vi "Autonomous Independent (Spencer Scott's conflicted copy 2017-03-24).vi"() -> ()   [LabVIEW 2016]
doc: "This VI is called when autonomous begins, and will automatically be terminated when autonomous ends. You can carry out timed or sensor driven robot movement independently without needing to return to the caller."
uses:
  Control 1.ctl
  <vilib>/Rock Robotics/Network Tables/NT Read String.vi
  <vilib>/Rock Robotics/Network Tables/NT Write String.vi
  Robot Global Data.vi
panel:
  in  "Drive PID":T1={"proportional gain (Kc)"=0.08, "integral time (Ti, min)"=0.0, "derivative time (Td, min)"=0.0} {"derivative time (Td, min)" format="%.3f"; "integral time (Ti, min)" format="%.3f"; "proportional gain (Kc)" format="%.3f"}
  # "Be sure to right-click and choose Data Operations>>Make Current Value default if you want to save the array values with the VI"
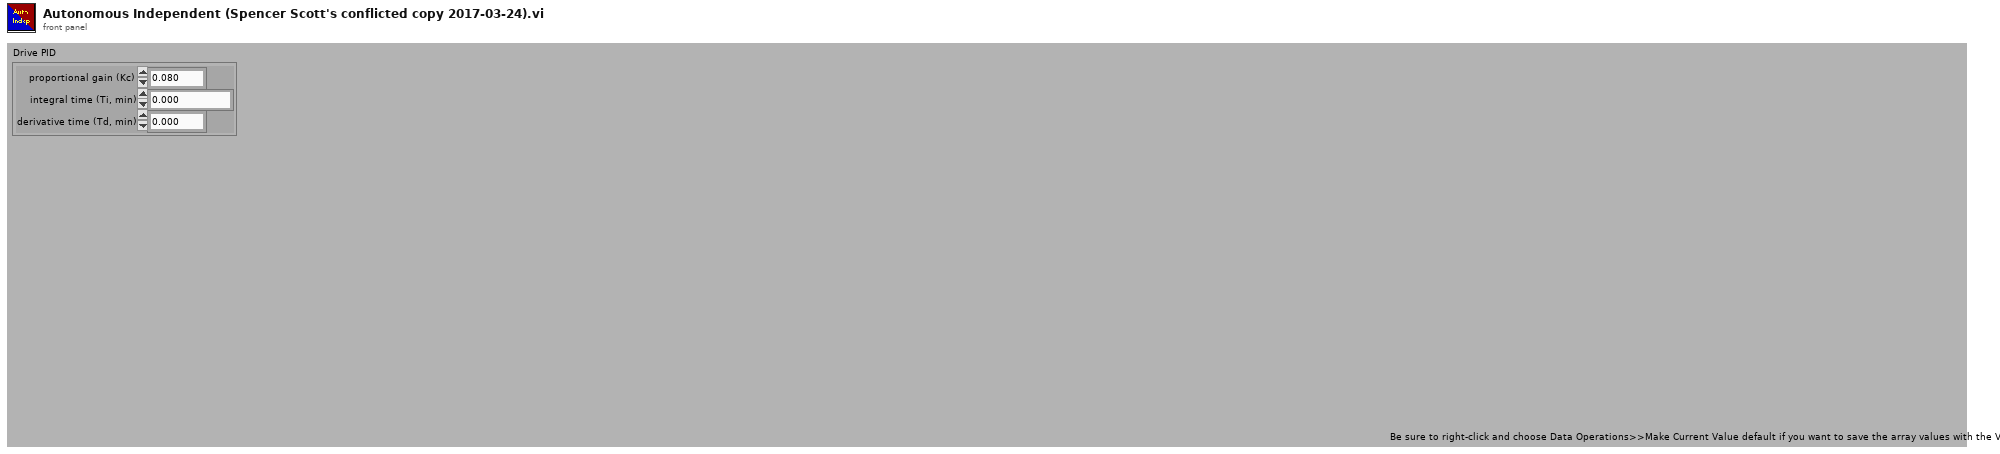
[diagram p1: front panel]
types:
  T1 = cluster{"proportional gain (Kc)":dbl, "integral time (Ti, min)":dbl, "derivative time (Td, min)":dbl}
  T2 = typedef "WPI_GyroDevRef.ctl" = cluster{"DevStatus":errorcluster, "Analog Channel":T3, "Offset":dbl, "Gain (VoltsPerDegree/Second)":dbl, "Gyro Type":enum16{"Analog", "XRS450"}, "Handle":i32, "SPI Bus":T4, "Device Found":bool, "Sample Rate":dbl, "Calibrate On Open":bool}
  T3 = typedef "FPGA_AIChannel.ctl" = enum8{"AI 0", "AI 1", "AI 2", "AI 3", "AI MXP 0", "AI MXP 1", "AI MXP 2", "AI MXP 3", "Invalid"}
  T4 = typedef "spi_bus.ctl" = enum16{"SPI On-Board, CS0", "SPI On-Board, CS1", "SPI On-Board, CS2", "SPI On-Board, CS3", "SPI MXP", "Invalid"}
  T5 = typedef "WPI_DriverStationAllianceInfo.ctl" = enum16{"Red", "Blue", "Invalid"}
  T6 = typedef "Control 1.ctl" = u32
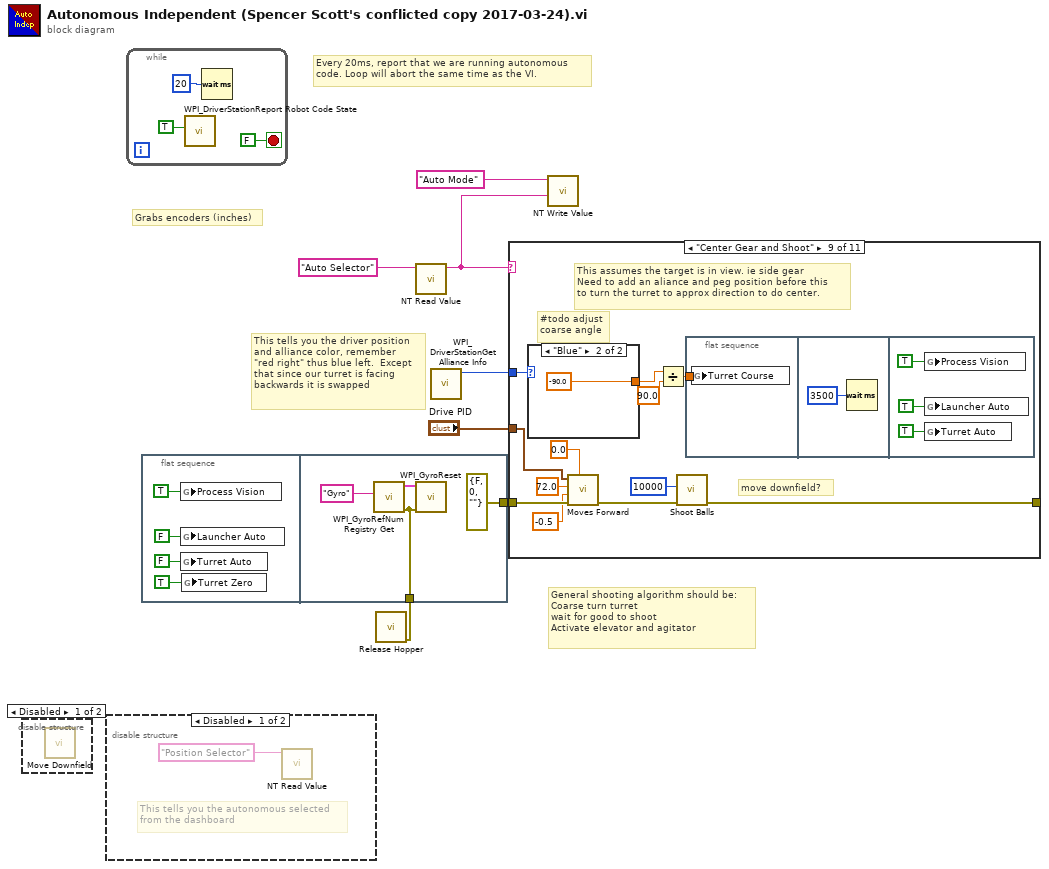
[diagram p0: block diagram]
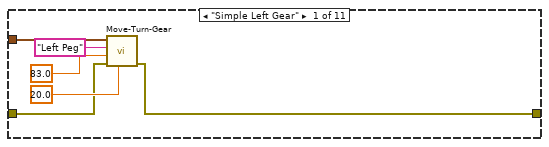
[diagram p4: hidden frame]
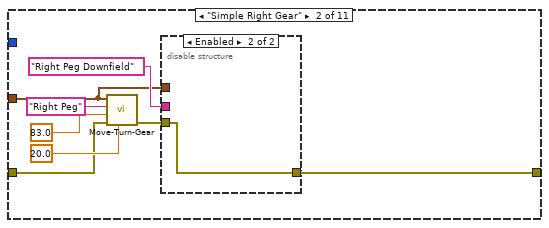
[diagram p5: hidden frame]
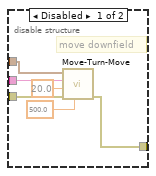
[diagram p6: hidden frame]
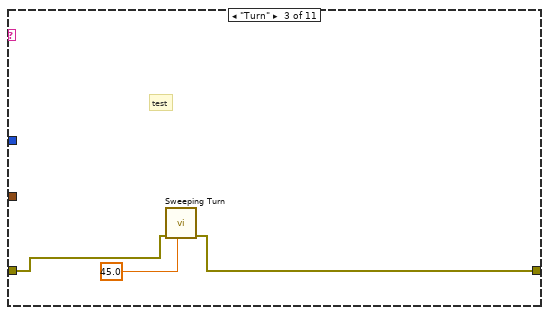
[diagram p7: hidden frame]
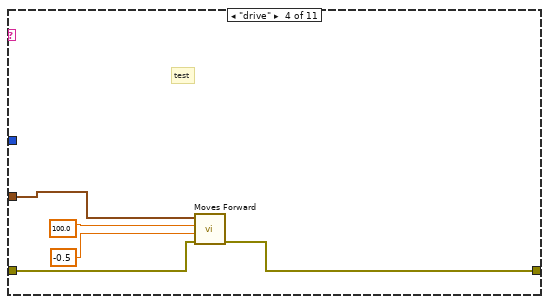
[diagram p8: hidden frame]
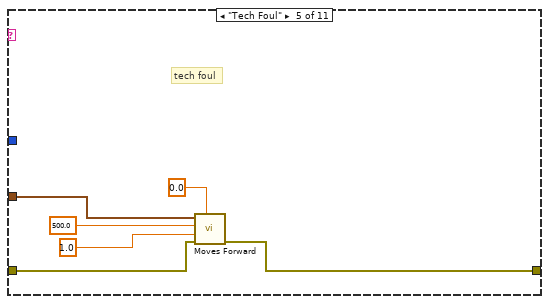
[diagram p9: hidden frame]
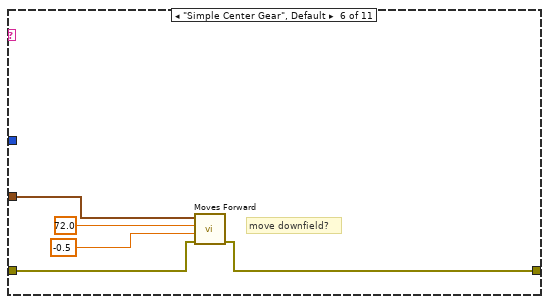
[diagram p10: hidden frame]
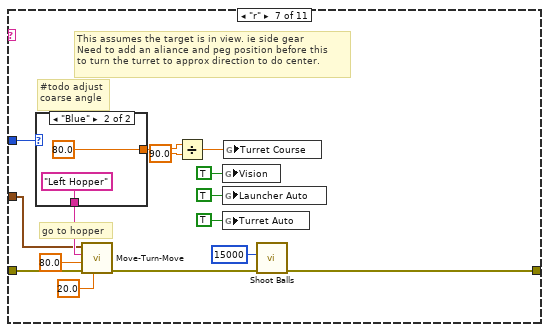
[diagram p11: hidden frame]
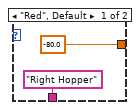
[diagram p12: hidden frame]
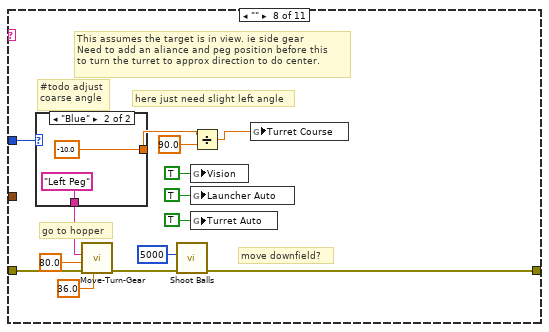
[diagram p13: hidden frame]
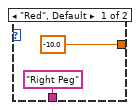
[diagram p14: hidden frame]
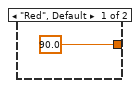
[diagram p15: hidden frame]
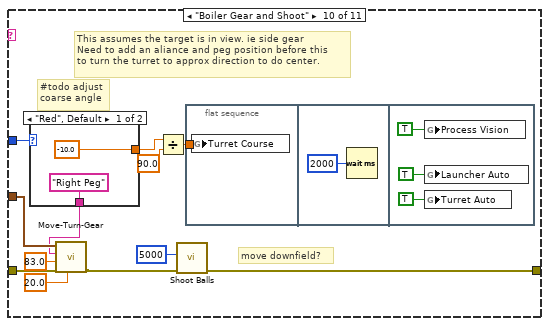
[diagram p16: hidden frame]
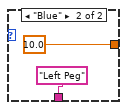
[diagram p17: hidden frame]
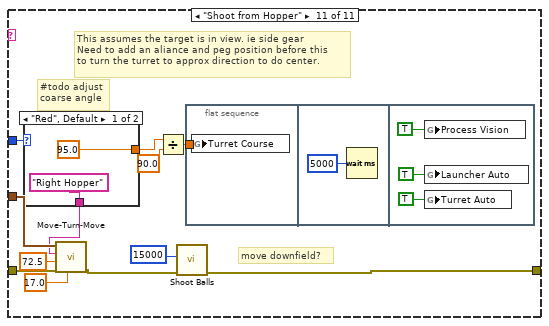
[diagram p18: hidden frame]
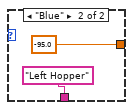
[diagram p19: hidden frame]
diagram:
  # "General shooting algorithm should be:\nCoarse turn turret\nwait for good to shoot\nActivate elevator and agitator"
  # "Every 20ms, report that we are running autonomous\ncode. Loop will abort the same time as the VI."
  # "This tells you the driver position\nand alliance color, remember\n\"red right\" thus blue left.  Except\nthat since our turret is facing\nbackwards it is swapped"
  # "Grabs encoders (inches)"
  n1 = disable-structure shown="Disabled" {
    frame Disabled {
      n2 = call "Move Downfield.vi"() -> ()  [unwired: 11 in, 1 out]
    }
    frame Enabled {
    }
  }
  n3 = disable-structure shown="Disabled" {
    frame Disabled {
      # "This tells you the autonomous selected\nfrom the dashboard"
      n4 = call-poly <vilib>:"NT Read Value.vi"("Name"="Position Selector") -> ()  [unwired: 9 in, 2 out]
    }
    frame Enabled {
    }
  }
  n5 = while {
    stop <- FALSE stop-if-true
    n6 = call <vilib>:"WPI_DriverStationReport Robot Code State.vi"("Autonomous"=TRUE) -> ()  [unwired: 10 in, 1 out]
    n7 = Wait (ms)(milliseconds to wait=u32 20) -> ()  [unwired: 1 out]
  }
  n8 = flat-sequence {
    tunnel: [w17] -> w3
    tunnel: [errorcluster {"status"=FALSE, "code"=0, "source"=""} ("error out")] -> w1
    frame #0 {
      n9 = global write "Robot Global Data.vi" "Process Vision"(TRUE ("Launcher Auto")) -> ()
      n10 = global write "Robot Global Data.vi" "Launcher Auto"(FALSE ("Launcher Auto")) -> ()
      n11 = global write "Robot Global Data.vi" "Turret Auto"(FALSE ("Launcher Auto")) -> ()
      n12 = global write "Robot Global Data.vi" "Turret Zero"(TRUE ("Launcher Auto")) -> ()
    }
    frame #1 {
      n13 = call <vilib>:"WPI_GyroRefNum Registry Get.vi"("refnum name"="Gyro") -> ("error out"=w17:errorcluster, "GyroDevRef"=w19:T2)  [unwired: 9 in]
      n14 = call <vilib>:"WPI_GyroReset.vi"("error in"=w17, "GyroDevRef"=w19) -> ()  [unwired: 8 in, 2 out]
    }
  }
  n15 = call "Release Hopper.vi"("error in (no error)"=w3) -> ()  [unwired: 10 in, 1 out]
  n16 = call-poly <vilib>:"NT Read Value.vi"("Name"="Auto Selector") -> ("String"=w4:string)  [unwired: 9 in, 1 out]
  n17 = call <vilib>:"WPI_DriverStationGet Alliance Info.vi"() -> ("Alliance"=w2:T5)  [unwired: 11 out]
  n18 = case shown="\"Center Gear and Shoot\"" w4 {
    tunnel: "Drive PID" -> [w21 w27 _ w47 w53 w58 w60 _ w100 w117 w138]
    tunnel: w1 -> [w23 w31 w41 w48 w54 w59 w74 w92 w105 w121 w142]
    tunnel: [w20 w26 w43 w44 w51 w55 w73 w91 w108 w127 w148] -> _
    tunnel: w2 -> [_ _ _ _ _ _ w66 w84 w107 w126 w147]
    frame "Simple Left Gear" {
      n19 = call "Move-Turn-Gear.vi"("toGear"=20.0, "error in (no error)"=w23, "gearDistance"=83.0, "Position"="Left Peg", "PID gains"=w21) -> ("error out"=w20:errorcluster)  [unwired: 6 in]
    }
    frame "Simple Right Gear" {
      n20 = call "Move-Turn-Gear.vi"("toGear"=20.0, "error in (no error)"=w31, "gearDistance"=83.0, "Position"="Right Peg", "PID gains"=w27) -> ("error out"=w29:errorcluster)  [unwired: 6 in]
      n21 = disable-structure shown="Enabled" {
        disable-tunnel: w29 -> [w39 w40]
        disable-tunnel: "Right Peg Downfield" ("Position") -> [w38 _]
        disable-tunnel: w27 -> [w37 _]
        disable-tunnel: [w36 w40] -> w26
        frame Disabled {
          # "move downfield"
          n22 = call "Move-Turn-Move.vi"("toGear"=500.0, "error in (no error)"=w39, "gearDistance"=20.0, "Position"=w38, "PID gains"=w37) -> ("error out"=w36:errorcluster)  [unwired: 6 in]
        }
        frame Enabled {
        }
      }
    }
    frame "Turn" {
      # "test"
      n23 = call "Sweeping Turn.vi"("upper angle limit"=45.0 ("upper limit"), "error in"=w41) -> ("error out"=w43:errorcluster)  [unwired: 9 in]
    }
    frame "drive" {
      # "test"
      n24 = call "Moves Forward.vi"("error in (no error)"=w48, "Speed"=-0.5, "forwardDistance"=100.0, "PID gains"=w47) -> ("error out"=w44:errorcluster)  [unwired: 5 in, 2 out]
    }
    frame "Tech Foul" {
      # "tech foul"
      n25 = call "Moves Forward.vi"("yaw setpoint"=0.0, "error in (no error)"=w54, "Speed"=1.0, "forwardDistance"=500.0, "PID gains"=w53) -> ("error out"=w51:errorcluster)  [unwired: 4 in, 2 out]
    }
    frame "Simple Center Gear", Default {
      # "move downfield?"
      n26 = call "Moves Forward.vi"("error in (no error)"=w59, "Speed"=-0.5, "forwardDistance"=72.0, "PID gains"=w58) -> ("error out"=w55:errorcluster)  [unwired: 5 in, 2 out]
    }
    frame "r" {
      # "#todo adjust\ncoarse angle"
      # "This assumes the target is in view. ie side gear\nNeed to add an aliance and peg position before this\nto turn the turret to approx direction to do center."
      # "go to hopper"
      n27 = case shown="\"Blue\"" w66 {
        tunnel: [-80.0 80.0] -> w65
        tunnel: ["Right Hopper" ("Name") "Left Hopper" ("Name")] -> w63
        frame "Red", Default {
        }
        frame "Blue" {
        }
      }
      n28 = call "Move-Turn-Move.vi"("toGear"=20.0, "error in (no error)"=w74, "gearDistance"=80.0, "Position"=w63, "PID gains"=w60) -> ("error out"=w72:errorcluster)  [unwired: 6 in]
      n29 = Divide(x=w65, y=90.0) -> (x/y=w62:dbl)
      n30 = global write "Robot Global Data.vi" "Vision"(TRUE ("Launcher Auto")) -> ()
      n31 = global write "Robot Global Data.vi" "Launcher Auto"(TRUE ("Launcher Auto")) -> ()
      n32 = global write "Robot Global Data.vi" "Turret Auto"(TRUE ("Launcher Auto")) -> ()
      n33 = global write "Robot Global Data.vi" "Turret Course"(w62) -> ()
      n34 = call "Shoot Balls.vi"("error in (no error)"=w72, "milliseconds to shoot"=u32 15000) -> ("error out"=w73:errorcluster)  [unwired: 9 in]
    }
    frame "" {
      # "move downfield?"
      # "here just need slight left angle"
      # "#todo adjust\ncoarse angle"
      # "This assumes the target is in view. ie side gear\nNeed to add an aliance and peg position before this\nto turn the turret to approx direction to do center."
      # "go to hopper"
      n35 = case shown="\"Blue\"" w84 {
        tunnel: [-10.0 -10.0] -> w81
        tunnel: ["Right Peg" ("Name") "Left Peg" ("Name")] -> w82
        frame "Red", Default {
        }
        frame "Blue" {
        }
      }
      n36 = call "Move-Turn-Gear.vi"("toGear"=36.0, "error in (no error)"=w92, "gearDistance"=80.0, "Position"=w82) -> ("error out"=w90:errorcluster)  [unwired: 7 in]
      n37 = call "Shoot Balls.vi"("error in (no error)"=w90, "milliseconds to shoot"=u32 5000) -> ("error out"=w91:errorcluster)  [unwired: 9 in]
      n38 = global write "Robot Global Data.vi" "Vision"(TRUE ("Launcher Auto")) -> ()
      n39 = global write "Robot Global Data.vi" "Launcher Auto"(TRUE ("Launcher Auto")) -> ()
      n40 = global write "Robot Global Data.vi" "Turret Auto"(TRUE ("Launcher Auto")) -> ()
      n41 = Divide(x=w81, y=90.0) -> (x/y=w80:dbl)
      n42 = global write "Robot Global Data.vi" "Turret Course"(w80) -> ()
    }
    frame "Center Gear and Shoot" {
      # "move downfield?"
      # "#todo adjust\ncoarse angle"
      # "This assumes the target is in view. ie side gear\nNeed to add an aliance and peg position before this\nto turn the turret to approx direction to do center."
      n43 = case shown="\"Blue\"" w107 {
        tunnel: [90.0 -90.0] -> w98
        frame "Red", Default {
        }
        frame "Blue" {
        }
      }
      n44 = call "Moves Forward.vi"("yaw setpoint"=0.0, "error in (no error)"=w105, "Speed"=-0.5, "forwardDistance"=72.0, "PID gains"=w100) -> ("error out"=w104:errorcluster)  [unwired: 4 in, 2 out]
      n45 = Divide(x=w98, y=90.0) -> (x/y=w99:dbl)
      n46 = call "Shoot Balls.vi"("error in (no error)"=w104, "milliseconds to shoot"=T6 10000) -> ("error out"=w108:errorcluster)  [unwired: 9 in]
      n47 = flat-sequence {
        tunnel: w99 -> [w109]
        frame #0 {
          n48 = global write "Robot Global Data.vi" "Turret Course"(w109) -> ()
        }
        frame #1 {
          n49 = Wait (ms)(milliseconds to wait=u32 3500) -> ()  [unwired: 1 out]
        }
        frame #2 {
          n50 = global write "Robot Global Data.vi" "Process Vision"(TRUE ("Launcher Auto")) -> ()
          n51 = global write "Robot Global Data.vi" "Launcher Auto"(TRUE ("Launcher Auto")) -> ()
          n52 = global write "Robot Global Data.vi" "Turret Auto"(TRUE ("Launcher Auto")) -> ()
        }
      }
    }
    frame "Boiler Gear and Shoot" {
      # "move downfield?"
      # "#todo adjust\ncoarse angle"
      # "This assumes the target is in view. ie side gear\nNeed to add an aliance and peg position before this\nto turn the turret to approx direction to do center."
      n53 = case shown="\"Red\", Default" w126 {
        tunnel: [-10.0 10.0] -> w123
        tunnel: ["Right Peg" ("refnum name") "Left Peg" ("refnum name")] -> w116
        frame "Red", Default {
        }
        frame "Blue" {
        }
      }
      n54 = call "Move-Turn-Gear.vi"("toGear"=20.0, "error in (no error)"=w121, "gearDistance"=83.0, "Position"=w116, "PID gains"=w117) -> ("error out"=w120:errorcluster)  [unwired: 6 in]
      n55 = Divide(x=w123, y=90.0) -> (x/y=w124:dbl)
      n56 = call "Shoot Balls.vi"("error in (no error)"=w120, "milliseconds to shoot"=u32 5000) -> ("error out"=w127:errorcluster)  [unwired: 9 in]
      n57 = flat-sequence {
        tunnel: w124 -> [w128]
        frame #0 {
          n58 = global write "Robot Global Data.vi" "Turret Course"(w128) -> ()
        }
        frame #1 {
          n59 = Wait (ms)(milliseconds to wait=u32 2000) -> ()  [unwired: 1 out]
        }
        frame #2 {
          n60 = global write "Robot Global Data.vi" "Process Vision"(TRUE ("Launcher Auto")) -> ()
          n61 = global write "Robot Global Data.vi" "Launcher Auto"(TRUE ("Launcher Auto")) -> ()
          n62 = global write "Robot Global Data.vi" "Turret Auto"(TRUE ("Launcher Auto")) -> ()
        }
      }
    }
    frame "Shoot from Hopper" {
      # "move downfield?"
      # "#todo adjust\ncoarse angle"
      # "This assumes the target is in view. ie side gear\nNeed to add an aliance and peg position before this\nto turn the turret to approx direction to do center."
      n63 = case shown="\"Red\", Default" w147 {
        tunnel: [95.0 -95.0] -> w144
        tunnel: ["Right Hopper" ("refnum name") "Left Hopper" ("refnum name")] -> w137
        frame "Red", Default {
        }
        frame "Blue" {
        }
      }
      n64 = call "Move-Turn-Move.vi"("toGear"=17.0, "error in (no error)"=w142, "gearDistance"=72.5, "Position"=w137, "PID gains"=w138) -> ("error out"=w141:errorcluster)  [unwired: 6 in]
      n65 = Divide(x=w144, y=90.0) -> (x/y=w145:dbl)
      n66 = call "Shoot Balls.vi"("error in (no error)"=w141, "milliseconds to shoot"=u32 15000) -> ("error out"=w148:errorcluster)  [unwired: 9 in]
      n67 = flat-sequence {
        tunnel: w145 -> [w149]
        frame #0 {
          n68 = global write "Robot Global Data.vi" "Turret Course"(w149) -> ()
        }
        frame #1 {
          n69 = Wait (ms)(milliseconds to wait=u32 5000) -> ()  [unwired: 1 out]
        }
        frame #2 {
          n70 = global write "Robot Global Data.vi" "Process Vision"(TRUE ("Launcher Auto")) -> ()
          n71 = global write "Robot Global Data.vi" "Launcher Auto"(TRUE ("Launcher Auto")) -> ()
          n72 = global write "Robot Global Data.vi" "Turret Auto"(TRUE ("Launcher Auto")) -> ()
        }
      }
    }
  }
  n73 = call-poly <vilib>:"NT Write Value.vi"("String"=w4, "Name"="Auto Mode" ("refnum name")) -> ()  [unwired: 9 in, 1 out]
